vi "Load plugin from absolute path.vi"(2 "error in (no error)":errorcluster, 3 "Absolute Path":path) -> (0 "error out":errorcluster, 1 "Generic Plugin out":refnum<class "Generic Plugin.lvclass">)   [LabVIEW 2020, in "Generic Plugin.lvclass"]
uses:
  Generic Plugin.lvclass
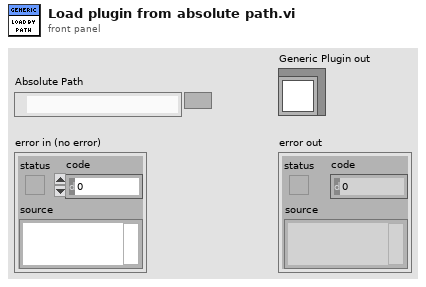
[diagram p1: front panel]
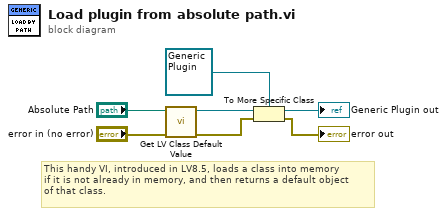
[diagram p0: block diagram]
diagram:
  # "This handy VI, introduced in LV8.5, loads a class into memory\nif it is not already in memory, and then returns a default object\nof that class."
  n1 = call <vilib>:"Get LV Class Default Value.vi"("error in (no error)"="error in (no error)", "class path"="Absolute Path") -> ("error out"=w4:errorcluster, "object"=w5:refnum<class>)  [unwired: 8 in]
  n2 = To More Specific Class(target class=refnum<class "Generic Plugin.lvclass"> refnum ("Generic Plugin.lvclass"), reference=w5, error in=w4) -> (specific class reference=→"Generic Plugin out":refnum<class "Generic Plugin.lvclass">, error out=→"error out":errorcluster)
